vi "Identificar_Switch_Presionado.vi"(10 "Get Response":string, 11 "Valor Actual":bool[](array[boolean])) -> (2 "number":u32, 3 "Switch Activado":bool[](array[boolean]))   [LabVIEW 2019]
uses:
  <vilib>/regexp/Match Regular Expression.xnode
panel:
  out "Sumar/Restar":bool[](array[boolean])
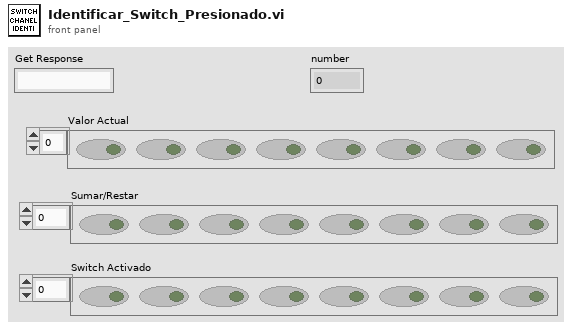
[diagram p1: front panel]
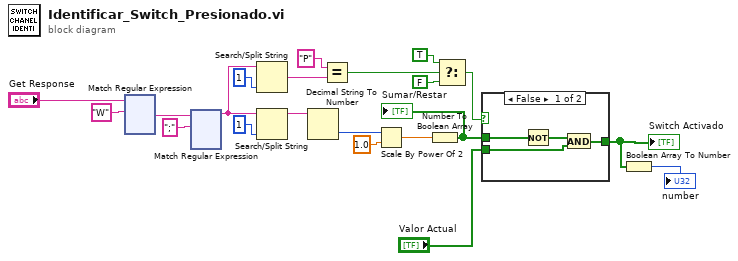
[diagram p0: block diagram]
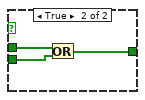
[diagram p2: hidden frame]
diagram:
  n1 = xnode "Match Regular Expression"("input string"="Get Response", "regular expression"="W") -> ("after match"=w17:string)  [unwired: 4 in, 4 out]
  n2 = xnode "Match Regular Expression"("input string"=w17, "regular expression"=";") -> ("before match"=w20:string)  [unwired: 4 in, 4 out]
  n3 = Search/Split String(string=w20, offset (0)=1) -> (match + rest of string=w14:string)  [unwired: 1 in, 2 out]
  n4 = Search/Split String(string=w20, offset (0)=1) -> (substring before match=w7:string)  [unwired: 1 in, 2 out]
  n5 = Decimal String To Number(string=w7) -> (number=w6:i32)  [unwired: 2 in, 1 out]
  n6 = Equal?(x="P", y=w14) -> (x = y?=w12:bool)
  n7 = Scale By Power Of 2(n=w6, x=1.0) -> (x*2^n=w9:dbl)
  n8 = Number To Boolean Array(number=w9) -> (Boolean array=w4:bool[])
  "Sumar/Restar" <- w4
  n9 = Select(t=TRUE, s=w12, f=FALSE) -> (s? t:f=w5:bool)
  n10 = case shown="False" w5 {
    tunnel: "Valor Actual" -> [w23 w28]
    tunnel: w4 -> [w25 w27]
    tunnel: [w22 w26] -> w2
    frame False {
      n11 = Not(x=w25) -> (.not. x?=w24:bool[])
      n12 = And(x=w24, y=w23) -> (x .and. y?=w22:bool[])
    }
    frame True {
      n13 = Or(x=w27, y=w28) -> (x .or. y?=w26:bool[])
    }
  }
  "Switch Activado" <- w2
  n14 = Boolean Array To Number(Boolean array=w2) -> (number=→"number":u32)
